vi "Log If Error.vi"(4 "Event Time":timestamp, 6 "Include Warnings(F)":bool, 7 "Event Level (Error)":T1=enum."Error", 8 "Error In":errorcluster, 9 "Clear After Logging?(F)":bool, 11 "SourceID":string) -> (0 "error out":errorcluster)   [LabVIEW 2019, in "Singleton Event Log.lvlib"]
uses:
  <vilib>/gpm_packages/@cs/event-logger/Source/Composed Log/Singleton Event Log/Singleton Event Log.lvlib
  <vilib>/gpm_packages/@cs/event-logger/Source/Composed Log/Types/Log Level.ctl
  <vilib>/gpm_packages/@cs/event-logger/Source/Composed Log/LoggerReference/LoggerReference.lvclass
  <vilib>/gpm_packages/@cs/event-logger/Source/Composed Log/Composed Log.lvlib
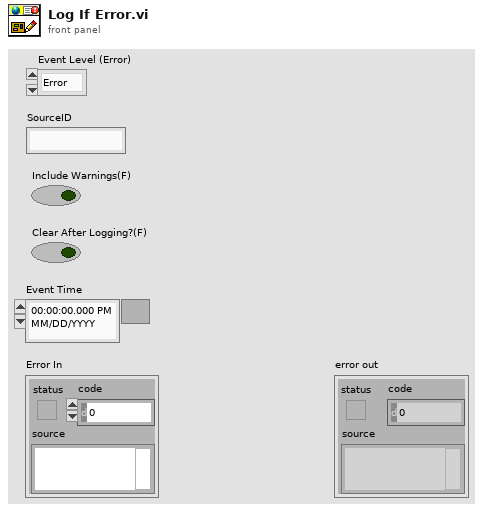
[diagram p1: front panel]
types:
  T1 = typedef "Composed Log.lvlib/Log Level.ctl" = enum16{"Debug", "Info", "Warning", "Error", "Critical"}
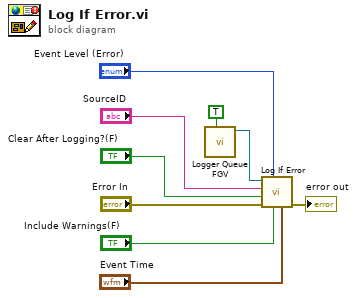
[diagram p0: block diagram]
diagram:
  n1 = call <vilib>:"Logger Queue FGV.vi"("Read?"=TRUE) -> ("LogReference Instance Out"=w8:refnum<class "LoggerReference.lvclass">)  [unwired: 10 in]
  n2 = call <vilib>:"Log If Error.vi"("Event Time"="Event Time", "Include Warnings(F)"="Include Warnings(F)", "Event Level (Error)"="Event Level (Error)", "Error In"="Error In", "Clear After Logging?(F)"="Clear After Logging?(F)", "SourceID"="SourceID", "Log Instance"=w8) -> ("error out"=→"error out":errorcluster)  [unwired: 3 in, 1 out]
